vi "Set Group UIs.vi"(8 "error in (no error)":errorcluster, 9 "Tx Group UI":refnum<class "User Interface.lvclass">, 10 "Rx Group UI":refnum<class "User Interface.lvclass">, 11 "Component UI in":refnum<class "Component User Interfaces.lvclass">) -> (0 "error out":errorcluster, 3 "Component UI out":refnum<class "Component User Interfaces.lvclass">)   [LabVIEW 2017, in "DSF Core.lvlib" / "Component User Interfaces.lvclass"]
uses:
  Component User Interfaces.lvclass
  User Interface/User Interface.lvclass
  Component User Interfaces.lvclass/Component User Interfaces.ctl
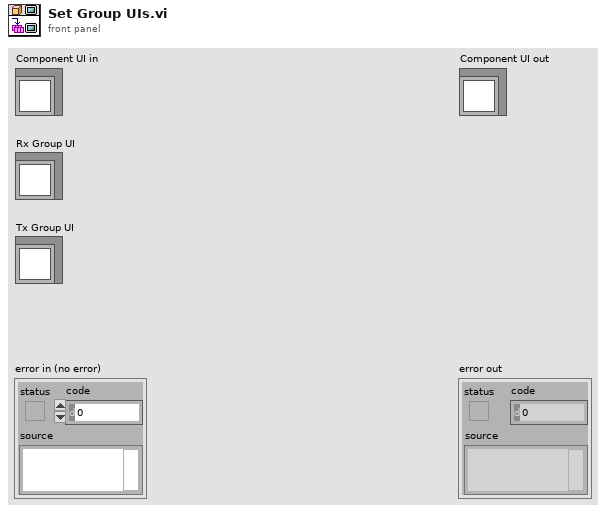
[diagram p1: front panel]
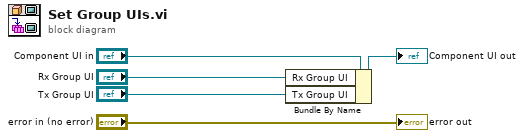
[diagram p0: block diagram]
diagram:
  n1 = Bundle By Name(cluster="Component UI in", "Rx Group UI"="Rx Group UI", "Tx Group UI"="Tx Group UI") -> (→"Component UI out":refnum<class "Component User Interfaces.lvclass">)
  "error out" <- "error in (no error)"
